vi "Write Camera State and try nr.vi"(9 "current try":u8, 10 "Camera State":T1=enum."Restart", 11 "Camera Actor in":refnum<class "Camera Actor.lvclass">) -> (3 "Camera Actor out":refnum<class "Camera Actor.lvclass">)   [LabVIEW 2014, in "Camera Actor.lvlib" / "Camera Actor.lvclass"]
uses:
  Camera Actor.lvclass
  Operation Mode.ctl
  Camera Actor.lvclass/Camera Actor.ctl
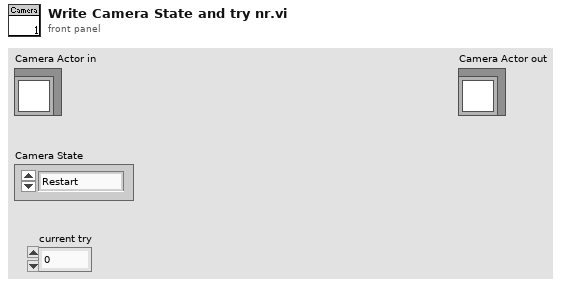
[diagram p1: front panel]
types:
  T1 = typedef "Camera Actor.lvlib/Camera Actor.lvclass/Operation Mode.ctl" = enum16{"Run", "Stop", "Exit", "Error", "Restart"}
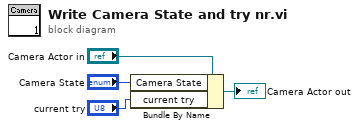
[diagram p0: block diagram]
diagram:
  n1 = Bundle By Name(cluster="Camera Actor in", "Camera State"="Camera State", "current try"="current try") -> (→"Camera Actor out":refnum<class "Camera Actor.lvclass">)
